vi "Monitor Errors.vi"(8 "error in (no error)":errorcluster, 11 "Mediator in":refnum<class "Mediator.lvclass">) -> (0 "error out":errorcluster, 2 "Sequence Error Info":T1, 3 "Mediator out":refnum<class "Mediator.lvclass">)   [LabVIEW 2015, in "Mediator.lvlib" / "Mediator.lvclass"]
doc: "This returns the error status of the most recent sequence executed by the Mediator. This VI blocks until sequence data is returned or the Mediator is shut down."
uses:
  Mediator.lvclass
  Controls/Sequence Return Info.ctl
  Mediator.lvclass/Mediator.ctl
  Sequence/Sequence.lvclass
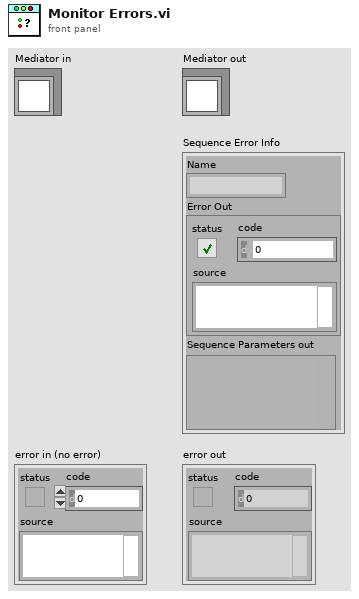
[diagram p1: front panel]
types:
  T1 = typedef "Mediator.lvlib/Sequence.lvclass/Sequence Return Info.ctl" = cluster{"Name":string, "Error Out":errorcluster, "Sequence Parameters out":variant}
  T2 = typedef "Mediator.lvlib/Sequence.lvclass/Sequence Error.ctl" = cluster{"Name":string, "Error Out":errorcluster, "Sequence Parameters out":variant}
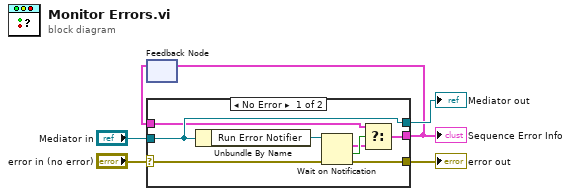
[diagram p0: block diagram]
diagram:
  n1 = feedback #1() -> (w1:T2)  [unwired: 1 in]
  n2 = case shown="No Error" "error in (no error)" {
    selector: "error in (no error)" -> [w12 w17]
    tunnel: [w11 w17] -> w5
    tunnel: [w14 w16] -> w3
    tunnel: "Mediator in" -> [w14 w16]
    tunnel: [w7 w15] -> w2
    tunnel: w1 -> [w9 w15]
    frame No Error {
      n3 = Unbundle By Name(w14) -> ("Run Error Notifier"=w13:refnum<notifier>)
      n4 = Wait on Notification(notifier=w13, error in (no error)=w12) -> (notification=w8:T2, timed out?=w10:bool, error out=w11:errorcluster)  [unwired: 2 in, 1 out]
      n5 = Select(t=w9, s=w10, f=w8) -> (s? t:f=w7:T2)
    }
    frame Error {
    }
  }
  "error out" <- w5
  "Mediator out" <- w3
  "Sequence Error Info" <- w2
  n6 = feedback-in #1(w2) -> ()
